vi "GT Get Crd Time.vi"(7 "fifo":i16, 8 "error in (no error)":errorcluster caption="错误输入（无错误）", 9 "pTime":T1, 10 "crd":i16, 11 "cardNum":i16) -> (0 "error out":errorcluster caption="错误输出", 1 "pTime out":T1, 3 "function return":i16)   [LabVIEW 2020, in "gts.lvlib"]
doc: "GT_API GT_GetCrdTime(short cardNum,short crd,TCrdTime *pTime,short fifo);"
uses:
  gts.lvlib
  dll/32bit/multi_card/gts.dll
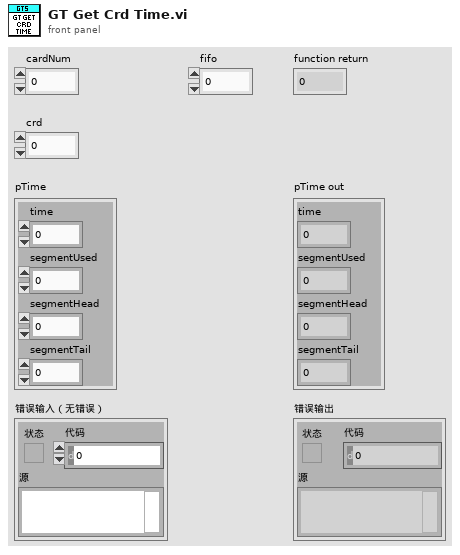
[diagram p1: front panel]
types:
  T1 = cluster{"time":dbl, "segmentUsed":i32, "segmentHead":i32, "segmentTail":i32}
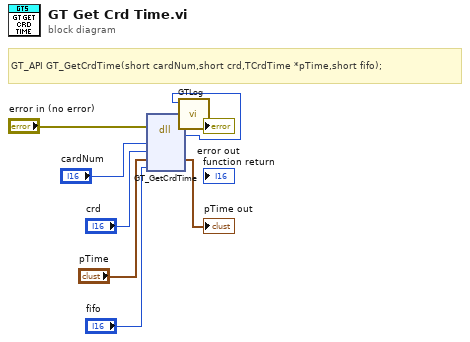
[diagram p0: block diagram]
diagram:
  # "GT_API GT_GetCrdTime(short cardNum,short crd,TCrdTime *pTime,short fifo);"
  n1 = dll-call lib="C:/1228/dll/32bit/multi_card/gts.dll" fn="GT_GetCrdTime"(error in="error in (no error)", "cardNum"="cardNum", "crd"="crd", "pTime"="pTime", "fifo"="fifo") -> (error out=w3:errorcluster, w1:i16, "pTime"=→"pTime out":T1)  [unwired: 5 in, 1 out]
  n2 = call "GTLog.vi"("error in (no error)"=w3, "Numeric"=w1) -> ("error out"=→"error out":errorcluster)  [unwired: 9 in]
